vi "async check errors.vi"(0 "module in":refnum<class "TBM module execution interface.lvclass">, 1 "fault handling":T1, 2 "configuration ref":refnum<data-value>, 3 "error fifo":refnum<k33>, 5 "previous error code in":i32, 9 "run flag in":u8, 11 "error in":errorcluster, 12 "engine error in":errorcluster) -> (4 "module out":refnum<class "TBM module execution interface.lvclass">, 6 "previous error code out":i32, 10 "run flag out":u8, 14 "engine error out":errorcluster, 15 "error out":errorcluster)   [LabVIEW 2013, in "main engine.lvlib"]
doc: "Checks for any errors which occurred in the module or in the process itself and performs the configured actions on behalf of the main engine. If necessary, it will pass the errors upstream to the engine for additional handling."
uses:
  main engine/main engine.lvlib
  main engine/fault handling spec.ctl
  Configuration/Error Actions.ctl
  Runtime/async error info.ctl
  <vilib>/NI/Tag Bus Module Framework/runtime/error classification.ctl
  <vilib>/NI/Tag Bus Module Framework/runtime/TBM module execution interface.lvclass
  <vilib>/NI/Tag Bus Module Framework/module configuration/TBM module configuration.lvclass
  Configuration/Standard Engine Configuration.lvclass
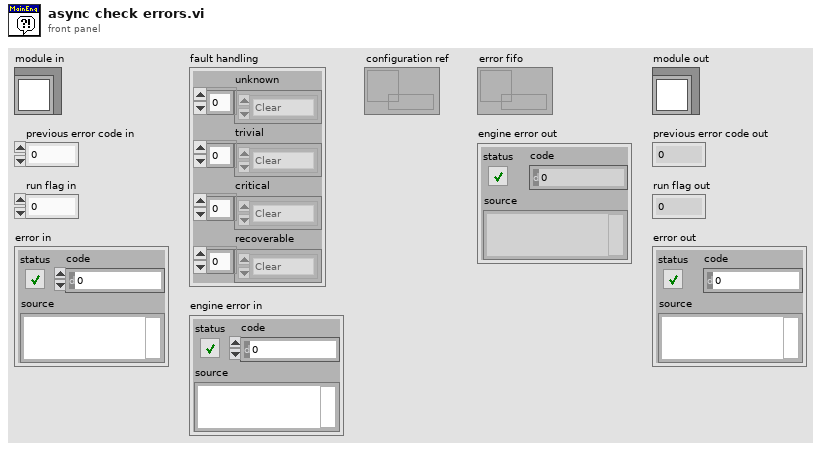
[diagram p1: front panel]
types:
  T1 = typedef "main engine.lvlib/fault handling spec.ctl" = cluster{"unknown":T2[], "trivial":T2[], "critical":T2[], "recoverable":T2[]}
  T2 = typedef "Standard Engine Configuration.lvclass/Error Actions.ctl" = enum16{"Clear", "Notify", "Log", "Stop Component", "Stop Engine", "Safe State", "Attempt Recovery"}
  T3 = typedef "main engine.lvlib/async error info.ctl" = cluster{"error code":i32, "error classification":T4}
  T4 = typedef "TBM module execution interface.lvclass/error classification.ctl" = enum16{"unknown", "none", "trivial", "recoverable", "critical"}
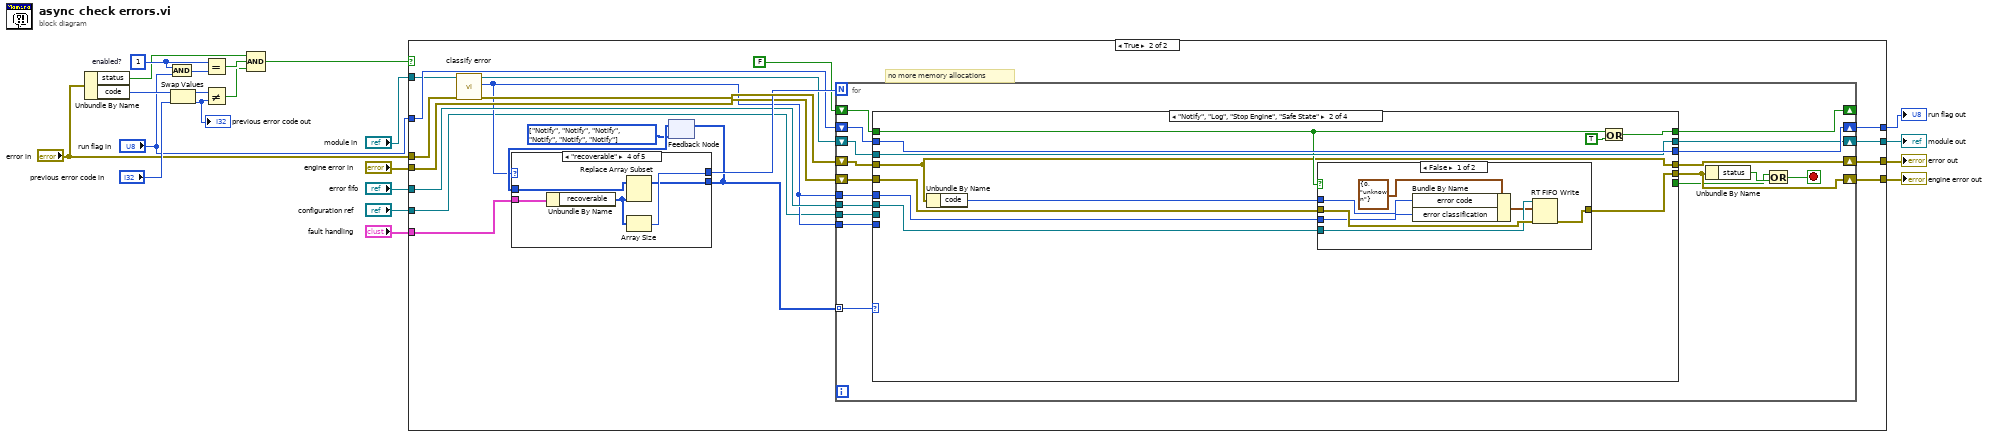
[diagram p0: block diagram]
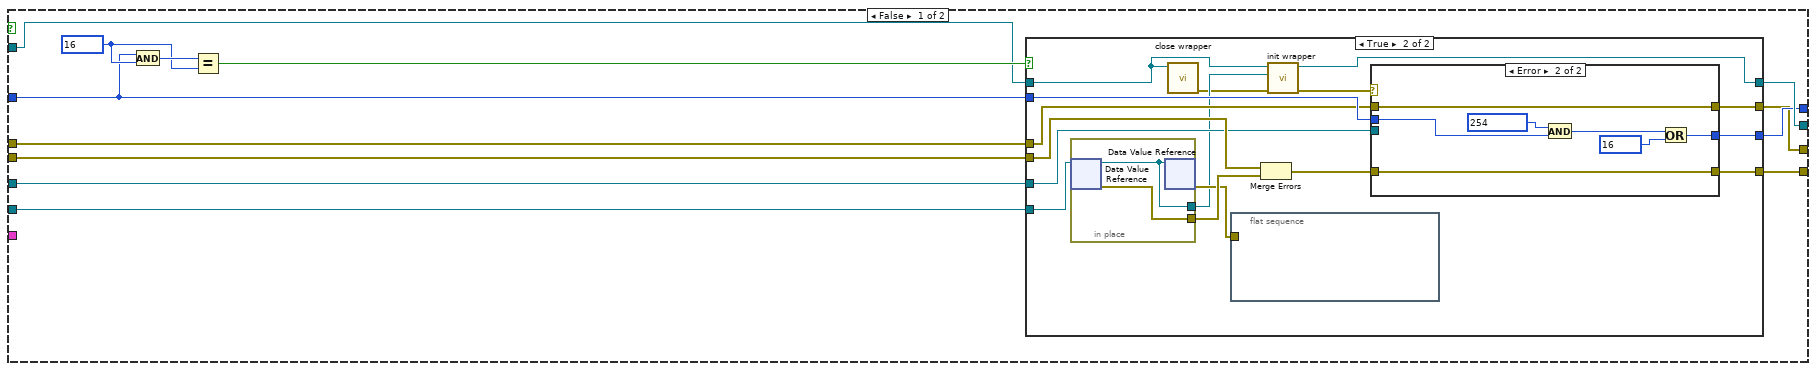
[diagram p2: hidden frame]
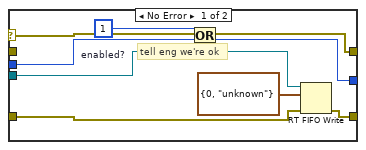
[diagram p4: hidden frame]
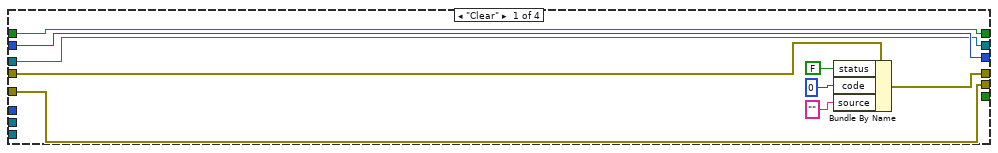
[diagram p5: hidden frame]
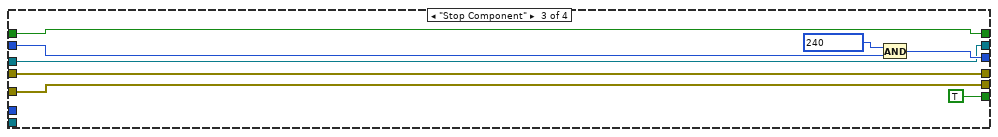
[diagram p7: hidden frame]
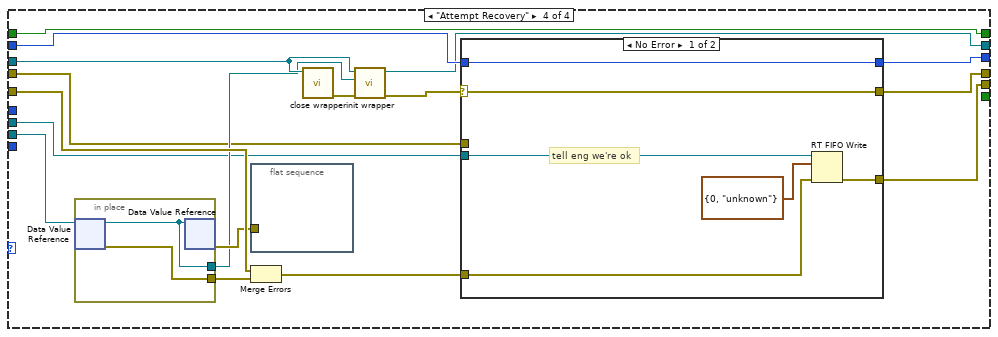
[diagram p8: hidden frame]
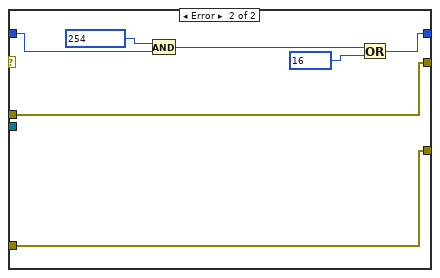
[diagram p9: hidden frame]
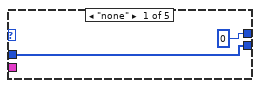
[diagram p10: hidden frame]
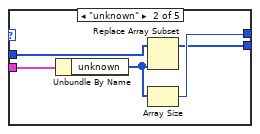
[diagram p11: hidden frame]
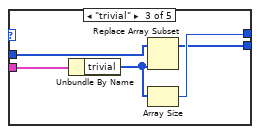
[diagram p12: hidden frame]
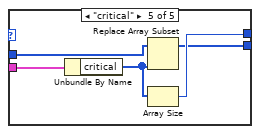
[diagram p13: hidden frame]
diagram:
  w17 = u8 1  # enabled?
  n1 = Unbundle By Name("error in") -> ("status"=w14:bool, "code"=w11:i32)
  n2 = And(x=w17, y="run flag in") -> (x .and. y?=w16:u8)
  n3 = Swap Values(12:w11, 14:"previous error code in") -> (1:w12:i32, 3:w8:i32)  [unwired: 1 in]
  "previous error code out" <- w8
  n4 = Equal?(x=w17, y=w16) -> (x = y?=w18:bool)
  n5 = Not Equal?(x=w12, y=w8) -> (x != y?=w13:bool)
  n6 = Compound Arithmetic op=AND(w14, w18, w13) -> (w15:bool)
  n7 = case shown="True" w15 {
    tunnel: "module in" -> [w31 w78]
    tunnel: [w30 w74] -> w9
    tunnel: "error in" -> [w25 w76]
    tunnel: [w24 w79] -> w10
    tunnel: "fault handling" -> [_ w85]
    tunnel: "run flag in" -> [w29 w82]
    tunnel: [w28 w80] -> w6
    tunnel: "engine error in" -> [w27 w83]
    tunnel: [w26 w81] -> w20
    tunnel: "error fifo" -> [w23 w84]
    tunnel: "configuration ref" -> [w22 w73]
    frame False {
      w33 = u8 16 ("x")
      n8 = And(x=w29, y=w33) -> (x .and. y?=w34:u8)
      n9 = Equal?(x=w34, y=w33) -> (x = y?=w32:bool)
      n10 = case shown="True" w32 {
        tunnel: w31 -> [w38 w54]
        tunnel: [w38 w46] -> w30
        tunnel: w29 -> [w37 w53]
        tunnel: [w37 w45] -> w28
        tunnel: w27 -> [w36 w51]
        tunnel: [w36 w48] -> w26
        tunnel: [w35 w47] -> w24
        tunnel: w25 -> [w35 w52]
        tunnel: w23 -> [_ w50]
        tunnel: w22 -> [_ w49]
        frame False {
          # "no recovery"
        }
        frame True {
          n11 = in-place {
            in-place-border: [w56] -> w43
            in-place-border: [w55] -> w41
            n12 = in-place-dvr #1(w49) -> (w55:refnum<class "TBM module configuration.lvclass">, w56:errorcluster)
            n13 = in-place-dvr #1(w55) -> (w42:errorcluster)  [unwired: 1 out]
          }
          n14 = call <vilib>:"close wrapper.vi"("module in"=w54) -> ("error out"=w39:errorcluster)  [unwired: 10 in]
          n15 = flat-sequence {
            tunnel: w42 -> [_]
            frame #0 {
            }
          }
          n16 = Merge Errors(w51, w43) -> (w40:errorcluster)
          n17 = call <vilib>:"init wrapper.vi"("error in (no error)"=w39, "module configuration"=w41, "module in"=w54) -> ("error out"=w44:errorcluster, "module out"=w46:refnum<class "TBM module execution interface.lvclass">)  [unwired: 5 in, 2 out]
          n18 = case shown="Error" w44 {
            selector: w44 -> [w59 _]
            tunnel: [w58 w69] -> w45
            tunnel: w53 -> [w64 w67]
            tunnel: w50 -> [w61 _]
            tunnel: [w62 w66] -> w48
            tunnel: w40 -> [w63 w66]
            tunnel: [w59 w65] -> w47
            tunnel: w52 -> [_ w65]
            frame No Error {
              w57 = u8 1  # enabled?
              # "tell eng we're ok"
              n19 = Or(x=w57, y=w64) -> (x .or. y?=w58:u8)
              n20 = RT FIFO Write(0:w61, 1:T3 {"error code"=0, "error classification"=enum."unknown"} ("element"), 3:w63) -> (11:w62:errorcluster)  [unwired: 2 in, 3 out]
            }
            frame Error {
              n21 = And(x=u8 254, y=w67) -> (x .and. y?=w71:u8)
              n22 = Or(x=w71, y=u8 16 ("x")) -> (x .or. y?=w69:u8)
            }
          }
        }
      }
    }
    frame True {
      w86 = T2[] [enum."Notify", enum."Notify", enum."Notify", enum."Notify", enum."Notify", enum."Notify"] items=["Clear", "Notify", "Log", "Stop Component", "Stop Engine", "Safe State", "Attempt Recovery"] ("critical")
      # "no more memory allocations"
      n23 = call-dynamic "classify error.vi"("error to classify"=w76, "module in"=w78) -> ("classified error"=w90:errorcluster, "error classification"=w77:T4, "module out"=w75:refnum<class "TBM module execution interface.lvclass">)  [unwired: 7 in]
      n24 = feedback #2(w86) -> (w87:T2[])
      n25 = case shown="\"recoverable\"" w77 {
        tunnel: w85 -> [_ w183 w188 w193 w198]
        tunnel: [w177 w180 w185 w190 w195] -> w88
        tunnel: [0 w182 w187 w192 w197] -> w89
        tunnel: w87 -> [w177 w181 w186 w191 w196]
        frame "none" {
        }
        frame "unknown" {
          n26 = Unbundle By Name(w183) -> ("unknown"=w179:T2[])
          n27 = Replace Array Subset(array=w181, new element=w179) -> (w180:T2[])  [unwired: 1 in]
          n28 = Array Size(array=w179) -> (size(s)=w182:i32)
        }
        frame "trivial" {
          n29 = Unbundle By Name(w188) -> ("trivial"=w184:T2[])
          n30 = Replace Array Subset(array=w186, new element=w184) -> (w185:T2[])  [unwired: 1 in]
          n31 = Array Size(array=w184) -> (size(s)=w187:i32)
        }
        frame "recoverable" {
          n32 = Unbundle By Name(w193) -> ("recoverable"=w189:T2[])
          n33 = Replace Array Subset(array=w191, new element=w189) -> (w190:T2[])  [unwired: 1 in]
          n34 = Array Size(array=w189) -> (size(s)=w192:i32)
        }
        frame "critical" {
          n35 = Unbundle By Name(w198) -> ("critical"=w194:T2[])
          n36 = Replace Array Subset(array=w196, new element=w194) -> (w195:T2[])  [unwired: 1 in]
          n37 = Array Size(array=w194) -> (size(s)=w197:i32)
        }
      }
      n38 = feedback-in #2(w88) -> ()
      n39 = for {
        N: w89 -> [_]
        shift-right: [w104] -> w80
        shift-left: w82 -> [w105]
        shift-right: [w106] -> w79
        shift-left: w90 -> [w107]
        tunnel: w84 -> [w101]
        tunnel: w88 -> [w108] mode=indexing
        shift-right: [w102] -> w81
        shift-left: w83 -> [w103]
        tunnel: w77 -> [w100]
        tunnel: w77 -> [w98]
        shift-right: [w96] -> w74
        shift-left: w75 -> [w97]
        tunnel: w73 -> [w95]
        shift-right: [w93] -> _
        shift-left: FALSE -> [w94]
        stop <- w92 stop-if-true
        n40 = case shown="\"Notify\", \"Log\", \"Stop Engine\", \"Safe State\"" w108 {
          tunnel: w107 -> [w117 w119 w144 w147]
          tunnel: [w114 w119 w144 w148] -> w106
          tunnel: w105 -> [w116 w128 w143 w160]
          tunnel: [w116 w128 w141 w161] -> w104
          tunnel: w103 -> [w115 w127 w142 w155]
          tunnel: [w115 w126 w142 w149] -> w102
          tunnel: w101 -> [_ w125 _ w151]
          tunnel: w100 -> [_ _ _ _]
          tunnel: w98 -> [_ w124 _ _]
          tunnel: w97 -> [w110 w123 w139 w159]
          tunnel: [w110 w123 w139 w158] -> w96
          tunnel: w95 -> [_ _ _ w156]
          tunnel: w94 -> [w109 w120 w138 w146]
          tunnel: [w109 w121 w138 w146] -> w93
          tunnel: [_ _ TRUE _] -> w91
          frame "Clear" {
            n41 = Bundle By Name(cluster=w117, "status"=FALSE, "code"=0, "source"="") -> (w114:errorcluster)
          }
          frame "Notify", "Log", "Stop Engine", "Safe State" {
            n42 = Unbundle By Name(w119) -> ("code"=w118:i32)
            n43 = case shown="False" w120 {
              tunnel: w127 -> [w135 w136]
              tunnel: [w134 w136] -> w126
              tunnel: w125 -> [w133 _]
              tunnel: w124 -> [w130 _]
              tunnel: w118 -> [w129 _]
              frame False {
                n44 = Bundle By Name(cluster=T3 {"error code"=0, "error classification"=enum."unknown"} ("element"), "error code"=w129, "error classification"=w130) -> (w131:T3)
                n45 = RT FIFO Write(0:w133, 1:w131, 3:w135) -> (11:w134:errorcluster)  [unwired: 2 in, 3 out]
              }
              frame True {
              }
            }
            n46 = Or(x=w120, y=TRUE) -> (x .or. y?=w121:bool)
          }
          frame "Stop Component" {
            n47 = And(x=u8 240, y=w143) -> (x .and. y?=w141:u8)
          }
          frame "Attempt Recovery" {
            n48 = in-place {
              in-place-border: [w163] -> w154
              in-place-border: [w162] -> w152
              n49 = in-place-dvr #3(w156) -> (w162:refnum<class "TBM module configuration.lvclass">, w163:errorcluster)
              n50 = in-place-dvr #3(w162) -> (w153:errorcluster)  [unwired: 1 out]
            }
            n51 = flat-sequence {
              tunnel: w153 -> [_]
              frame #0 {
              }
            }
            n52 = Merge Errors(w155, w154) -> (w150:errorcluster)
            n53 = call <vilib>:"close wrapper.vi"("module in"=w159) -> ("error out"=w145:errorcluster)  [unwired: 10 in]
            n54 = call <vilib>:"init wrapper.vi"("error in (no error)"=w145, "module configuration"=w152, "module in"=w159) -> ("error out"=w157:errorcluster, "module out"=w158:refnum<class "TBM module execution interface.lvclass">)  [unwired: 5 in, 2 out]
            n55 = case shown="No Error" w157 {
              selector: w157 -> [w164 _]
              tunnel: [w169 w174] -> w161
              tunnel: w160 -> [w169 w172]
              tunnel: w151 -> [w166 _]
              tunnel: [w167 w171] -> w149
              tunnel: w150 -> [w168 w171]
              tunnel: [w164 w170] -> w148
              tunnel: w147 -> [_ w170]
              frame No Error {
                # "tell eng we're ok"
                n56 = RT FIFO Write(0:w166, 1:T3 {"error code"=0, "error classification"=enum."unknown"} ("element"), 3:w168) -> (11:w167:errorcluster)  [unwired: 2 in, 3 out]
              }
              frame Error {
                n57 = And(x=u8 254, y=w172) -> (x .and. y?=w176:u8)
                n58 = Or(x=w176, y=u8 16 ("x")) -> (x .or. y?=w174:u8)
              }
            }
          }
        }
        n59 = Unbundle By Name(w102) -> ("status"=w99:bool)
        n60 = Or(x=w91, y=w99) -> (x .or. y?=w92:bool)
      }
    }
  }
  "run flag out" <- w6
  "error out" <- w10
  "module out" <- w9
  "engine error out" <- w20
